vi "solar_excel Worksheet Build (tsv).vi"(10 "Worksheets Cells":cluster{"Cells":string[][]}[](array[cluster]), 11 "Worksheets":string[](array[string])) -> (3 "Tab Delimited String":string)   [LabVIEW 2018]
doc: "This build a tab delimited text file separated by sections (i.e. '[MySheet1]').\n\n[MySheet1]\nA\\tB\\tC\nD\\tE\\tF\n[MySheet2]\n1\\t2\\t3\n4\\t5\\t6"
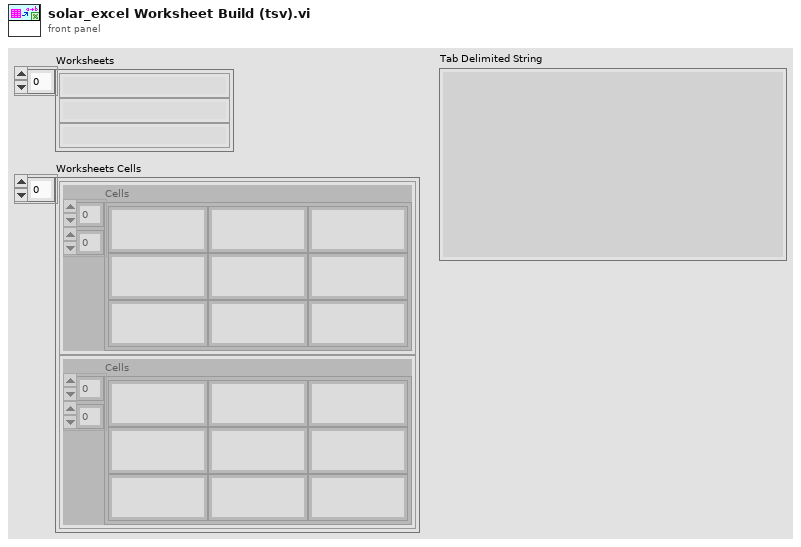
[diagram p1: front panel]
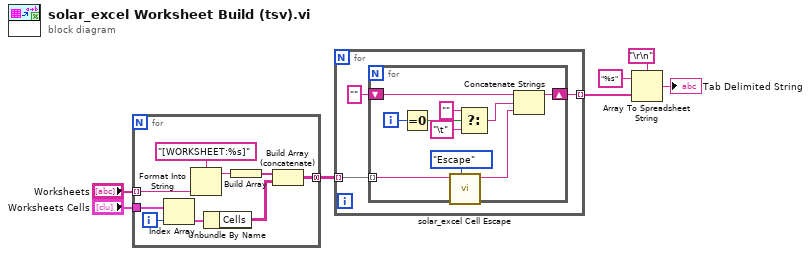
[diagram p0: block diagram]
diagram:
  n1 = for {
    tunnel: "Worksheets" -> [w13] mode=indexing
    tunnel: "Worksheets Cells" -> [w16]
    tunnel: [w8] -> w3 mode=concatenating
    i -> [w15]
    n2 = Index Array(array=w16, index=w15) -> (element=w12:cluster{"Cells":string[][]})
    n3 = Format Into String(format string="[WORKSHEET:%s]", w13) -> (resulting string=w11:string)  [unwired: 2 in, 1 out]
    n4 = Unbundle By Name(w12) -> ("Cells"=w9:string[][])
    n5 = Build Array(w11) -> (w10:string[])
    n6 = Build Array (concatenate)(w10, w9) -> (w8:string[][])
  }
  n7 = for {
    tunnel: w3 -> [w19] mode=indexing
    tunnel: [w17] -> w7 mode=indexing
    n8 = for {
      tunnel: w19 -> [w23] mode=indexing
      shift-right: [w27] -> w17
      shift-left: "" -> [w29]
      i -> [w26]
      n9 = Equal To 0?(x=w26) -> (x = 0?=w25:bool)
      n10 = call "solar_excel Cell Escape.vi"("Action (Escape)"=enum8{"Escape", "Unescape"}."Escape", "String in"=w23) -> ("String out"=w21:string)  [unwired: 9 in]
      n11 = Select(t="", s=w25, f="\t" ("Delimiter (\\t)")) -> (s? t:f=w28:string)
      n12 = Concatenate Strings(w29, w28, w21) -> (w27:string)
    }
  }
  n13 = Array To Spreadsheet String(delimiter (Tab)="\r\n", array=w7, 3:"%s" ("format string")) -> (spreadsheet string=→"Tab Delimited String":string)
